vi "record_wav.vi"() -> ()   [LabVIEW 2023]
uses:
  <vilib>/sound2/lvsound2.llb/Sound Data Format.ctl
panel:
  in  "sound format":T1={"sample rate (S/s)"=44100.0, "number of channels"=1, "bits per sample"=16}
  in  "Duration (s)":dbl=5.0
  in  "path":path
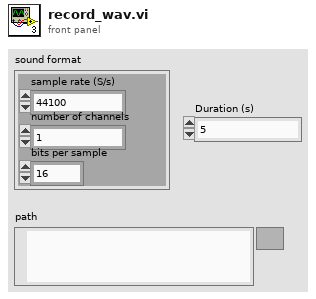
[diagram p1: front panel]
types:
  T1 = typedef "Sound Data Format.ctl" = cluster{"sample rate (S/s)":dbl, "number of channels":i32, "bits per sample":i32}
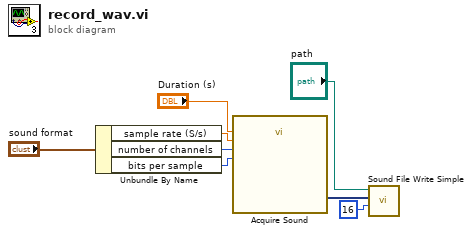
[diagram p0: block diagram]
diagram:
  n1 = Unbundle By Name("sound format") -> ("sample rate (S/s)"=w4:dbl, "number of channels"=w2:i32, "bits per sample"=w1:i32)
  n2 = call "Acquire Sound"("Duration (s)"="Duration (s)", "Sample rate (Hz)"=w4, "#Channels"=w2, "Resolution (bits)"=w1) -> ("Data"=w5:dynamicdata)  [unwired: 14 in, 1 out]
  n3 = call <vilib>:"Sound File Write Simple.vi"("bits per sample"=16, "data"=w5, "path"="path") -> ()  [unwired: 7 in, 2 out]
